vi "clLabview_blockUncompress.vi"(11 "vi_lib.lvlib:clFileReader.lvclass":refnum<class "clFileReader.lvclass">) -> (0 "return vale":i32, 3 "vi_lib.lvlib:clFileReader.lvclass 2":refnum<class "clFileReader.lvclass">)   [LabVIEW 2020, in "vi_lib.lvlib" / "clLabview.lvclass"]
uses:
  clLabview.lvclass
  clFileReader/clFileReader.lvclass
  clFile/clFile.lvclass
  zlib.dll
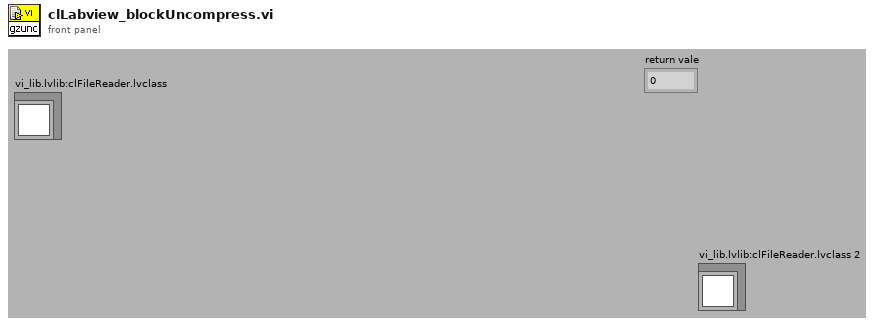
[diagram p1: front panel]
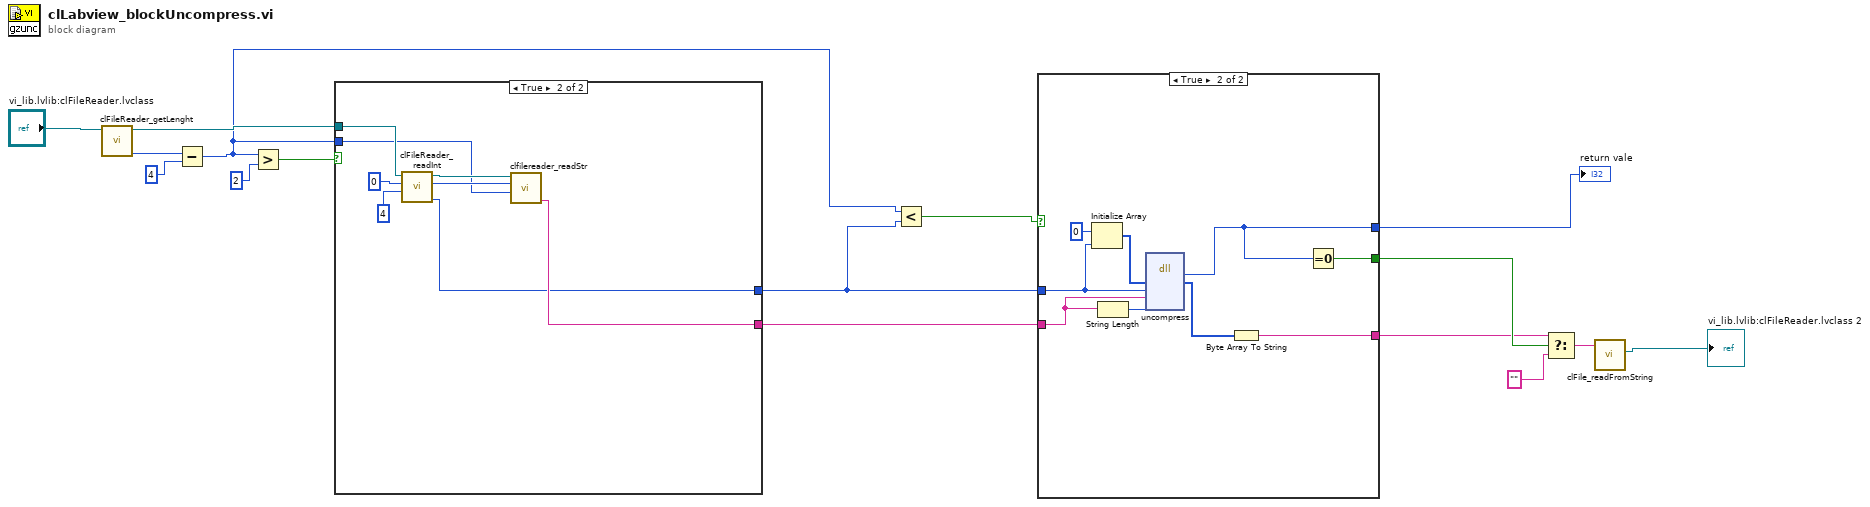
[diagram p0: block diagram]
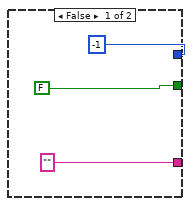
[diagram p2: hidden frame]
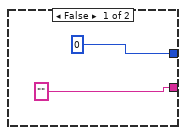
[diagram p3: hidden frame]
diagram:
  n1 = call "clFileReader_getLenght.vi"("clFileReader.lvclass IN"="vi_lib.lvlib:clFileReader.lvclass") -> ("blocklen"=w3:u32, "clFileReader.lvclassOut"=w13:refnum<class "clFileReader.lvclass">)  [unwired: 9 out]
  n2 = Subtract(x=w3, y=u32 4) -> (x-y=w2:u32)
  n3 = Greater?(x=w2, y=u32 2) -> (0:w14:bool)
  n4 = case shown="True" w14 {
    tunnel: w13 -> [_ w26]
    tunnel: w2 -> [_ w23]
    tunnel: ["" ("dest") w22] -> w8
    tunnel: [u32 0 ("OUT Value") w21] -> w6
    frame False {
    }
    frame True {
      n5 = call "clFileReader_readInt.vi"("size"=u32 4 ("offset"), "offset"=u32 0, "clFileReader.lvclass IN"=w26) -> ("OUT Value"=w21:u32, "new offset"=w24:u32, "clFileReader.lvclass OUT"=w25:refnum<class "clFileReader.lvclass">)  [unwired: 6 out]
      n6 = call "clfilereader_readStr.vi"("size"=w23, "offset"=w24, "clFileReader.lvclass IN"=w25) -> ("ReadStr - OUT Value"=w22:string)  [unwired: 8 out]
    }
  }
  n7 = Less?(x=w2, y=w6) -> (x < y?=w7:bool)
  n8 = case shown="True" w7 {
    tunnel: [FALSE w38] -> w10
    tunnel: ["" ("dest") w30] -> w9
    tunnel: w8 -> [_ w35]
    tunnel: w6 -> [_ w32]
    tunnel: [-1 ("return vale") w37] -> w5
    frame False {
    }
    frame True {
      n9 = Initialize Array(u8 0 ("element"), w32) -> (w34:u8[])
      n10 = String Length(string=w35) -> (length=w36:i32)
      n11 = dll-call lib="C:/Projets/Others/VI-Explorer-VI/zlib.dll" fn="uncompress"("dest"=w34, "dest_size"=w32, "src"=w35, "src_size"=w36) -> ("return vale"=w37:i32, "dest"=w31:u8[])  [unwired: 6 in, 2 out]
      n12 = Byte Array To String(unsigned byte array=w31) -> (string=w30:string)
      n13 = Equal To 0?(x=w37) -> (x = 0?=w38:bool)
    }
  }
  "return vale" <- w5
  n14 = Select(t=w9, s=w10, f="") -> (s? t:f=w12:string)
  n15 = call "clFile_readFromString.vi"("String"=w12) -> ("clFileReader.lvclass"=→"vi_lib.lvlib:clFileReader.lvclass 2":refnum<class "clFileReader.lvclass">)  [unwired: 10 out]
